vi "未命名 2 (子VI).vi"(9 "min distance":dbl, 10 "max distance":dbl, 11 "distance":dbl) -> (1 "b":dbl, 2 "g":dbl, 3 "r":dbl)   [LabVIEW 2012]
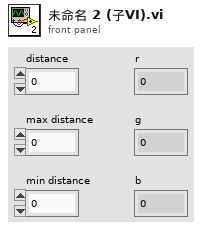
[diagram p1: front panel]
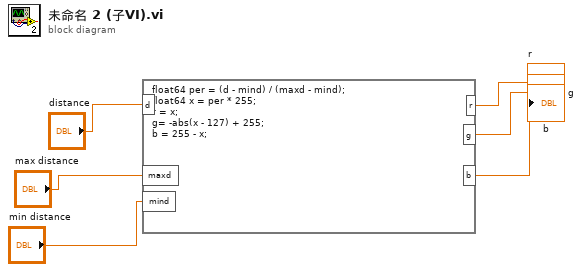
[diagram p0: block diagram]
diagram:
  n1 = formula code="float64 per = (d - mind) / (maxd - mind);\nfloat64 x = per * 255;\nr = x;\ng= -abs(x - 127) + 255;\nb = 255 - x;"("d"="distance", "maxd"="max distance", "mind"="min distance") -> ("r"=→"r":dbl, "g"=→"g":dbl, "b"=→"b":dbl)
